vi "Lookup Tag Values.vi"(8 "error in (no error)":errorcluster, 11 "Tag Expr in":refnum<class "Tag Expr.lvclass">) -> (0 "error out":errorcluster, 3 "Tag Expr out":refnum<class "Tag Expr.lvclass">)   [LabVIEW 2020, in "Tag Expr.lvclass"]
doc: "Lookup the current values of all Tags within the expression.\n\nValues are coerced to DBL type.\n\nSupported types are for Coercion are:\n- Boolean\n- Signed Integer\n- Unsigned Integer\n- Floating Point\n- String (with period decimal point)\n- Timestamp\n\nAll other types will return NaN with error 5605 reported."
uses:
  Tag Expr.lvclass
  C:/Program Files (x86)/National Instruments/LabVIEW 2020/vi.lib/LAVA/muParser/mupExpr/mupExpr.lvclass
  Tag Expr.lvclass/Tag Expr.ctl
  Tag/Tag.lvclass/Tag.ctl
  <vilib>/LAVA/muParser/mupExpr/mupExpr.lvclass/mupExpr.ctl
  <vilib>/LAVA/muParser/mupExpr/Set_MultiVar_Value.vi
  Tag/Read Value.vi
  Tag/Read Timestamp.vi
  <vilib>/LAVA/muParser/mupExpr/SetVarVal.vi
  <vilib>/LAVA/muParser/mupLib/mupSetVarValue.vi
  <vilib>/Utility/error.llb/Error Cluster From Error Code.vi
  <vilib>/ErrorRing/Error Ring.xnode
  <vilib>/LAVA/muParser/mupExpr/mupExpr.lvclass
  Core/Tag Core.lvclass
  C:/Users/leonidas/Documents/GitHub/tag-engine/Tag Expr/Tag Expr.lvclass
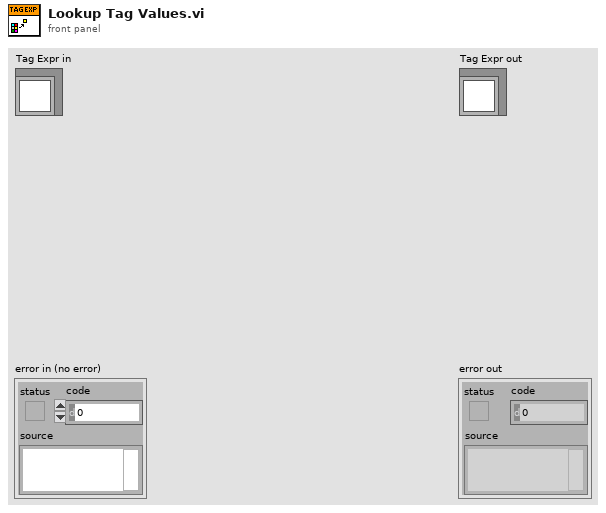
[diagram p1: front panel]
types:
  T1 = typedef "NI_Data Type.lvlib/Data Type.ctl" = enum8{"Invalid Type", "Void", "I8", "I16", "I32", "I64", "U8", "U16", "U32", "U64", "Single Float", "Double Float", "Extended Float", "Single Complex", "Double Complex", "Extended Complex", "Enum U8", "Enum U16", "Enum U32", "Enum U64", "Single Float With Unit", "Double Float With Unit", "Extended Float With Unit", "Single Complex with Unit", "Double Complex with Unit", "Extended Complex with Unit", "Boolean", "String", "Path", "Picture", "Tag", "Array", "Cluster", "Variant", "LV Variant", "Waveform", "Timestamp", "Digital Waveform", "Digital Data", "ExpressData", "Refnum", "External Data", "VI", "Poly VI", "LabVIEW Class Instance", "Fixed Point", "Set Collection", "Map Collection"}
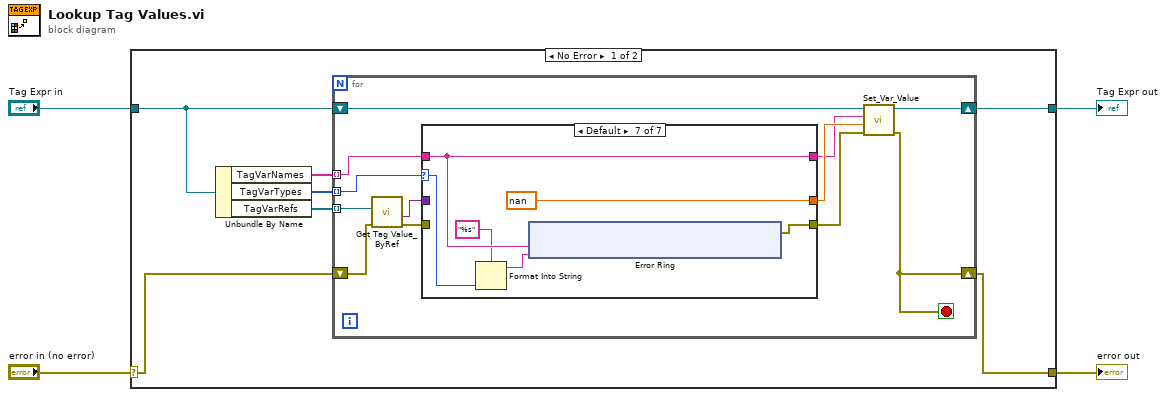
[diagram p0: block diagram]
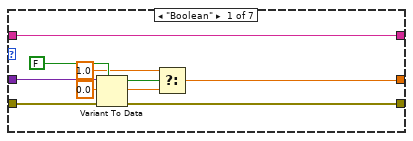
[diagram p2: hidden frame]
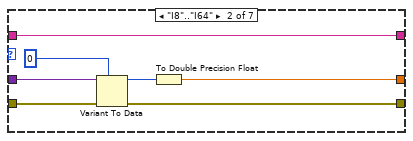
[diagram p3: hidden frame]
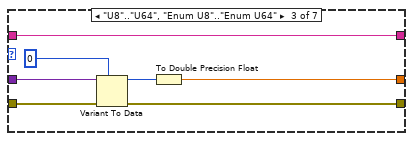
[diagram p4: hidden frame]
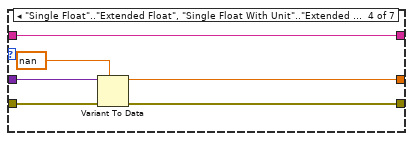
[diagram p5: hidden frame]
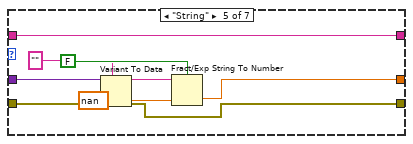
[diagram p6: hidden frame]
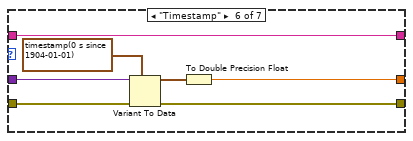
[diagram p7: hidden frame]
diagram:
  n1 = case shown="No Error" "error in (no error)" {
    selector: "error in (no error)" -> [w6 w84]
    tunnel: [w5 w84] -> w3
    tunnel: [w9 w83] -> w1
    tunnel: "Tag Expr in" -> [w10 w83]
    frame No Error {
      n2 = Unbundle By Name(w10) -> ("TagVarNames"=w7:string[], "TagVarTypes"=w8:T1[], "TagVarRefs"=w11:refnum<data-value>[])
      n3 = for {
        tunnel: w11 -> [w23] mode=indexing
        shift-right: [w18] -> w9
        shift-left: w10 -> [w19]
        tunnel: w8 -> [w20] mode=indexing
        tunnel: w7 -> [w13] mode=indexing
        shift-right: [w15] -> w5
        shift-left: w6 -> [w17]
        stop <- w15 stop-if-true
        n4 = call "Get Tag Value_ByRef.vi"("error in (no error)"=w17, "Tag Ref in"=w23) -> ("error out"=w22:errorcluster, "Value"=w21:variant)  [unwired: 6 in, 2 out]
        n5 = case shown="Default" w20 {
          selector: w20 -> [_ _ _ _ _ _ w70]
          tunnel: w21 -> [w32 w39 w46 w52 w60 w68 _]
          tunnel: [w27 w36 w43 w50 w56 w64 nan ("f")] -> w14
          tunnel: [w26 w34 w41 w48 w54 w63 w73] -> w16
          tunnel: w22 -> [w25 w35 w42 w49 w55 w67 _]
          tunnel: w13 -> [w24 w33 w40 w47 w53 w62 w72]
          tunnel: [w24 w33 w40 w47 w53 w62 w72] -> w12
          frame "Boolean" {
            n6 = Variant To Data(error in=w25, type=FALSE, Variant=w32) -> (data=w30:bool, error out=w26:errorcluster)
            n7 = Select(t=1.0, s=w30, f=0.0) -> (s? t:f=w27:dbl)
          }
          frame "I8".."I64" {
            n8 = Variant To Data(error in=w35, type=i64 0, Variant=w39) -> (data=w37:i64, error out=w34:errorcluster)
            n9 = To Double Precision Float(number=w37) -> (double precision float=w36:dbl)
          }
          frame "U8".."U64", "Enum U8".."Enum U64" {
            n10 = Variant To Data(error in=w42, type=u64 0, Variant=w46) -> (data=w44:u64, error out=w41:errorcluster)
            n11 = To Double Precision Float(number=w44) -> (double precision float=w43:dbl)
          }
          frame "Single Float".."Extended Float", "Single Float With Unit".."Extended Float With Unit", "Fixed Point" {
            n12 = Variant To Data(error in=w49, type=nan, Variant=w52) -> (data=w50:dbl, error out=w48:errorcluster)
          }
          frame "String" {
            n13 = Variant To Data(error in=w55, type="", Variant=w60) -> (data=w58:string, error out=w54:errorcluster)
            n14 = Fract/Exp String To Number(use system decimal point (T)=FALSE, string=w58, default (0 dbl)=nan ("default (0 DBL)")) -> (number=w56:dbl)  [unwired: 1 in, 1 out]
          }
          frame "Timestamp" {
            n15 = Variant To Data(error in=w67, type=timestamp(0 s since 1904-01-01), Variant=w68) -> (data=w65:timestamp, error out=w63:errorcluster)
            n16 = To Double Precision Float(number=w65) -> (double precision float=w64:dbl)
          }
          frame Default {
            n17 = Format Into String(format string="%s", w70) -> (resulting string=w69:string)  [unwired: 2 in, 1 out]
            n18 = xnode "Error Ring"("parameter 0"=w72, "parameter 1"=w69) -> ("error out"=w73:errorcluster)
          }
        }
        n19 = call-poly <vilib>:"Set_Var_Value.vi"("error in (no error)"=w16, "varValue"=w14, "varName"=w12, "muExpr in"=w19) -> ("error out"=w15:errorcluster, "muExpr out"=w18:refnum<class "Tag Expr.lvclass">)  [unwired: 6 in]
      }
    }
    frame Error {
    }
  }
  "error out" <- w3
  "Tag Expr out" <- w1
